vi "aula 2.vi"() -> ()   [LabVIEW 2026]
panel:
  in  "Numeric 3":dbl
  out "°C 2":dbl(slide) scale=0.0..300.0
  out "x*y 2":dbl
  out "Numeric 2":i32
  in  "stop 2":bool
  in  "°F 2":dbl(slide) scale=0.0..300.0
  in  "Boolean":bool
  in  "stop":bool
  out "Numeric":i32
  out "x*y":dbl
  out "°C":dbl(slide) scale=0.0..300.0
  in  "°F":dbl(slide) scale=0.0..300.0
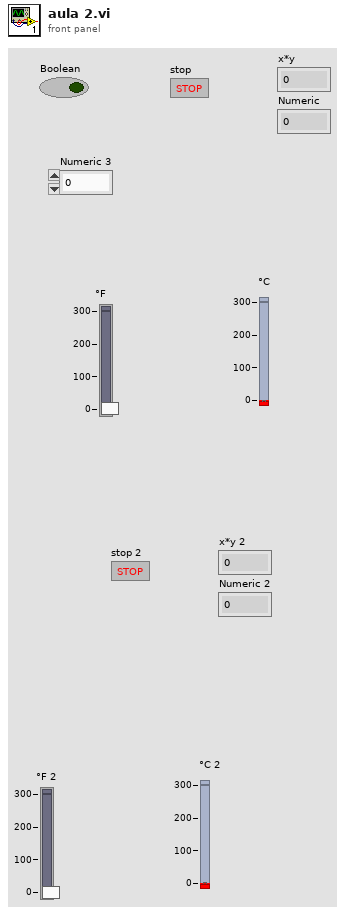
[diagram p1: front panel]
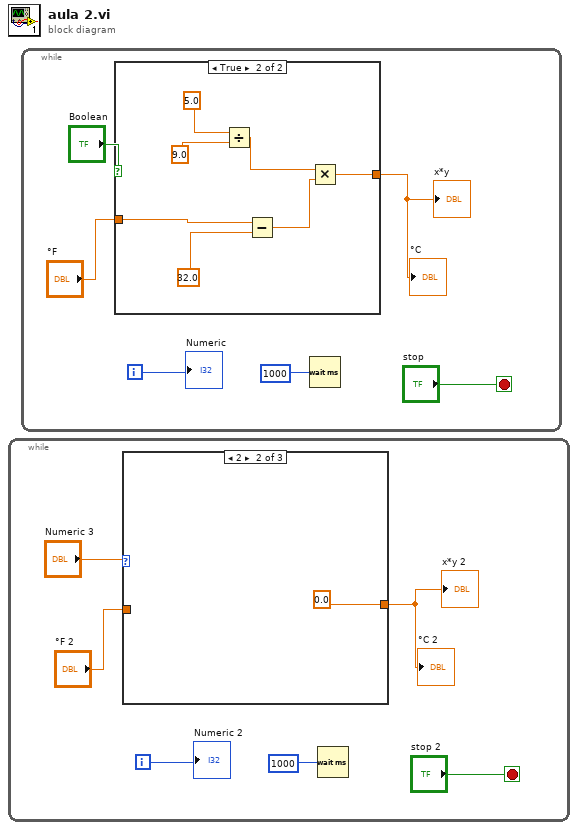
[diagram p0: block diagram]
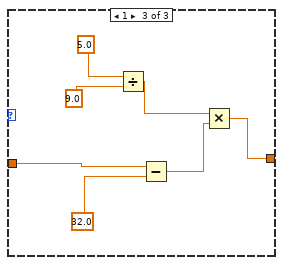
[diagram p3: hidden frame]
diagram:
  n1 = while {
    i -> [w5]
    stop <- "stop 2" stop-if-true
    n2 = case shown="2" "Numeric 3" {
      tunnel: [w7 0.0 ("°F 2") w10] -> w6
      tunnel: "°F 2" -> [w7 _ w9]
      frame 0, Default {
      }
      frame 2 {
      }
      frame 1 {
        n3 = Divide(x=5.0, y=9.0) -> (x/y=w13:dbl)
        n4 = Subtract(x=w9, y=32.0) -> (x-y=w14:dbl)
        n5 = Multiply(x=w13, y=w14) -> (x*y=w10:dbl)
      }
    }
    "°C 2" <- w6
    "x*y 2" <- w6
    n6 = Wait (ms)(milliseconds to wait=u32 1000) -> ()  [unwired: 1 out]
    "Numeric 2" <- w5
  }
  n7 = while {
    i -> [w20]
    stop <- "stop" stop-if-true
    n8 = case shown="True" "Boolean" {
      tunnel: [w22 w24] -> w21
      tunnel: "°F" -> [w22 w23]
      frame False {
      }
      frame True {
        n9 = Divide(x=5.0, y=9.0) -> (x/y=w27:dbl)
        n10 = Subtract(x=w23, y=32.0) -> (x-y=w28:dbl)
        n11 = Multiply(x=w27, y=w28) -> (x*y=w24:dbl)
      }
    }
    "°C" <- w21
    "x*y" <- w21
    n12 = Wait (ms)(milliseconds to wait=u32 1000) -> ()  [unwired: 1 out]
    "Numeric" <- w20
  }
